vi "Read configuration.vi"(8 "error in (no error)":errorcluster, 11 "Instrument Device in":refnum<class "Synchronization Instrument.lvclass">) -> (0 "error out":errorcluster, 2 "configuration":refnum<class "CEF_serializable configuration.lvclass">, 3 "Instrument Device out":refnum<class "Synchronization Instrument.lvclass">)   [LabVIEW 2025, in "Synchronization.lvlib" / "Synchronization Instrument.lvclass"]
uses:
  Synchronization Instrument.lvclass
  Users/Public/Documents/Sandia National Labs/TSS Plugin/CEF.lvlibp/serializable configuration/CEF_serializable configuration.lvclass
  Synchronization Instrument.lvclass/Synchronization Instrument.ctl
  Synchronization configuration/Synchronization configuration.lvclass
  C:/Users/Public/Documents/Sandia National Labs/TSS Plugin/CEF.lvlibp/serializable configuration/CEF_serializable configuration.lvclass
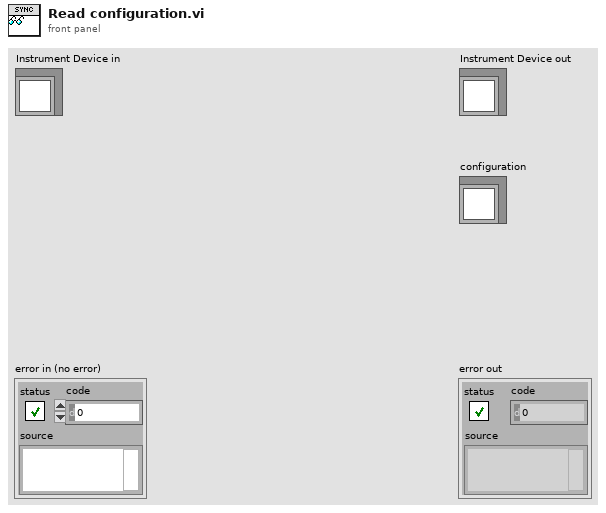
[diagram p1: front panel]
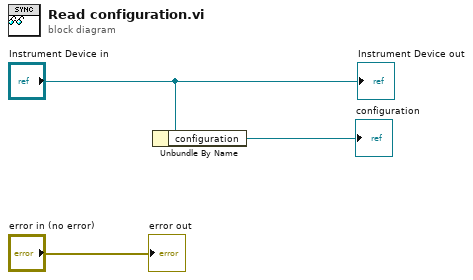
[diagram p0: block diagram]
diagram:
  n1 = Unbundle By Name("Instrument Device in") -> ("configuration"=→"configuration":refnum<class "Synchronization configuration.lvclass">)
  "error out" <- "error in (no error)"
  "Instrument Device out" <- "Instrument Device in"
